vi "Wait for Hot.vi"() -> ()   [LabVIEW 2013]
uses:
  Robot Global Data.vi
panel:
  in  "Move Speed":dbl=1.0
  in  "Move Duration (ms)":u32=1000
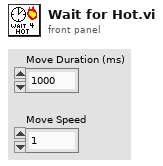
[diagram p1: front panel]
types:
  T1 = enum16{"Hold", "Pick Up", "Catch", "Aim", "Shoot", "Joystick"}
  T2 = enum16{"Hold", "Pick Up", "Catch", "Aim", "Shoot"}
  T3 = typedef "WPI_DriverStationMatch Info.ctl" = cluster{"Autonomous Elapsed Seconds":dbl, "TeleOp Elapsed Seconds":dbl, "Disabled Elapsed Seconds":dbl, "Visited Autonomous":bool, "Visited TeleOp":bool, "Visited Disabled":bool, "Autonomous Settings":cluster{"Autonomous Style":enum16{"Iterative", "Independent"}, "VI Refnum":refnum<vi>}}
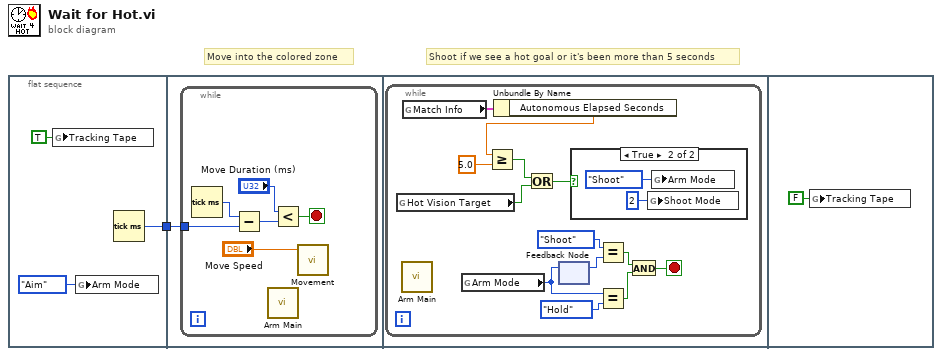
[diagram p0: block diagram]
diagram:
  # "Shoot if we see a hot goal or it's been more than 5 seconds"
  # "Move into the colored zone"
  n1 = flat-sequence {
    tunnel: [w3] -> w1
    tunnel: w1 -> [w5]
    frame #0 {
      n2 = global write "Robot Global Data.vi" "Tracking Tape"(TRUE ("Enable Vision")) -> ()
      n3 = global write "Robot Global Data.vi" "Arm Mode"(T1."Aim" ("Arm Mode")) -> ()
      n4 = Tick Count (ms)() -> (millisecond timer value=w3:u32)
    }
    frame #1 {
      n5 = while {
        tunnel: w5 -> [w10]
        stop <- w6 stop-if-true
        n6 = Tick Count (ms)() -> (millisecond timer value=w11:u32)
        n7 = Subtract(x=w11, y=w10) -> (x-y=w9:u32)
        n8 = call "Arm Main.vi"() -> ()  [unwired: 1 in]
        n9 = Less?(x="Move Duration (ms)", y=w9) -> (x < y?=w6:bool)
        n10 = call "Movement.vi"("Forward Speed"="Move Speed") -> ()  [unwired: 2 in]
      }
    }
    frame #2 {
    }
    frame #3 {
      n11 = global write "Robot Global Data.vi" "Tracking Tape"(FALSE ("Enable Vision")) -> ()
    }
  }
  n12 = while {
    stop <- w19 stop-if-true
    n13 = global read "Robot Global Data.vi" "Hot Vision Target"() -> (w24:bool)
    n14 = call "Arm Main.vi"() -> ()  [unwired: 1 in]
    n15 = global read "Robot Global Data.vi" "Match Info"() -> (w25:T3)
    n16 = global read "Robot Global Data.vi" "Arm Mode"() -> (w13:T2)
    n17 = Unbundle By Name(w25) -> ("Autonomous Elapsed Seconds"=w20:dbl)
    n18 = Greater Or Equal?(x=w20, y=5.0) -> (x >= y?=w23:bool)
    n19 = Or(x=w23, y=w24) -> (x .or. y?=w21:bool)
    n20 = feedback #1() -> (w14:T2)  [unwired: 1 in]
    n21 = feedback-in #1(w13) -> ()
    n22 = case shown="True" w21 {
      frame False {
      }
      frame True {
        n23 = global write "Robot Global Data.vi" "Shoot Mode"(i8 2 ("Shoot Mode")) -> ()
        n24 = global write "Robot Global Data.vi" "Arm Mode"(T1."Shoot" ("Arm Mode")) -> ()
      }
    }
    n25 = Equal?(x=T2."Shoot", y=w14) -> (x = y?=w16:bool)
    n26 = Equal?(x=w13, y=T1."Hold" ("Arm Mode")) -> (x = y?=w18:bool)
    n27 = And(x=w16, y=w18) -> (x .and. y?=w19:bool)
  }
